vi "SetPiePlot.vi"(0 "reference in":refnum<class "HTMLPlot.lvclass">, 1 "PiePlot.PlotLabels":string[](array[string]), 2 "Dataset":dbl[][](array[numeric]), 3 "DatasetLabels":string[](array[string]), 5 "error in (no error)":errorcluster, 6 "DoughnutStyle":bool, 7 "PlotColours":u32[](array[colorbox])) -> (14 "reference out":refnum<class "HTMLPlot.lvclass">, 19 "error out":errorcluster)   [LabVIEW 2019, in "HTMLPlot.lvclass"]
uses:
  HTMLPlot.lvclass
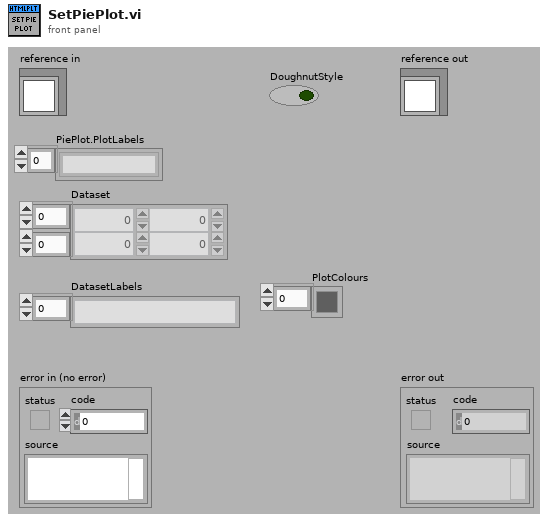
[diagram p1: front panel]
types:
  T1 = typedef "HTMLPlot.lvclass/ObjectAttributes.ctl" = cluster{"Attribute1":dbl, "GraphContainer":refnum<k7>, "ChartScriptFile":string, "UtilScriptFile(demoData)":string, "BaseHTML":string, "GenericProperties":cluster{"PlotType":T2, "PlotTitle":string, "XLabel":string, "YLabel":string, "ShowToolTip":bool}, "LegendProperties":cluster{"Show":bool, "Position":T3}, "BarPlot":cluster{"Dataset":dbl[][], "DatasetLabels":string[], "XLabels":string[], "PlotColours":u32[], "Stacked":bool}, "PiePlot":cluster{"Dataset":dbl[][], "DatasetLabels":string[], "PlotColours":u32[], "DoughnutStyle":bool, "PlotLabels":string[]}, "connection ID":refnum<k5>, "PortID":u64}
  T2 = typedef "HTMLPlot.lvclass/PlotType.ctl" = enum16{"bar", "line", "pie"}
  T3 = typedef "HTMLPlot.lvclass/LegendPosition.ctl" = enum16{"top", "right", "left", "bottom"}
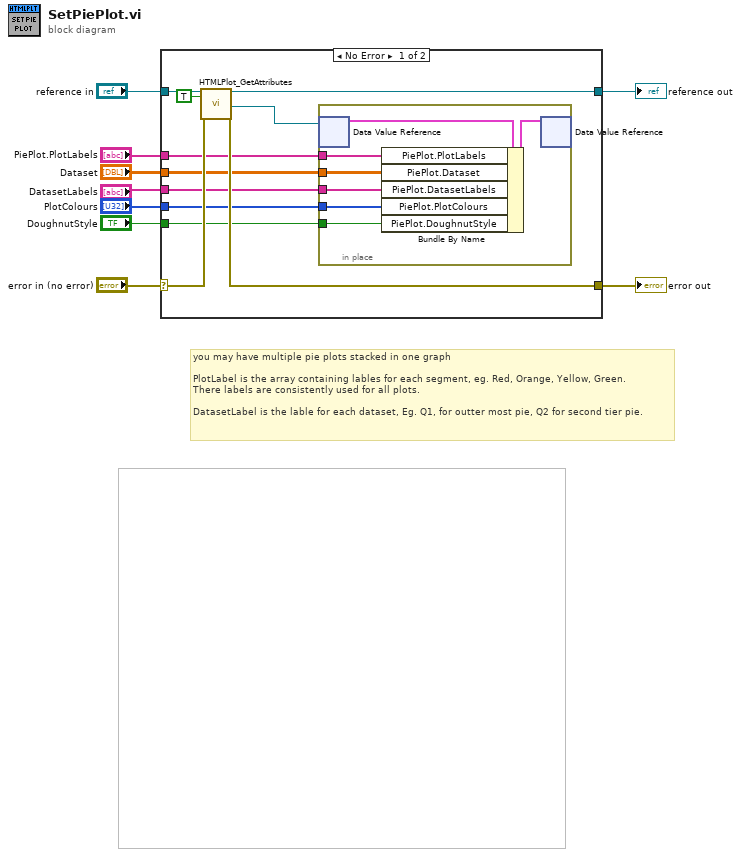
[diagram p0: block diagram]
diagram:
  # "you may have multiple pie plots stacked in one graph\n\nPlotLabel is the array containing lables for each segment, eg. Red, Orange, Yellow, Green.\nThere labels are consistently used for all plots.\n\nDatasetLabel is the lable for each dataset, Eg. Q1, for outter most pie, Q2 for second tier pie."
  n1 = case shown="No Error" "error in (no error)" {
    selector: "error in (no error)" -> [w20 w29]
    tunnel: [w19 w29] -> w8
    tunnel: [w17 w28] -> w6
    tunnel: "reference in" -> [w18 w28]
    tunnel: "Dataset" -> [w14 _]
    tunnel: "PlotColours" -> [w13 _]
    tunnel: "DatasetLabels" -> [w12 _]
    tunnel: "DoughnutStyle" -> [w11 _]
    tunnel: "PiePlot.PlotLabels" -> [w10 _]
    frame No Error {
      n2 = call "HTMLPlot_GetAttributes.vi"("reference in"=w18, "OnlyGetDvrReference(False)"=TRUE, "error in (no error)"=w20) -> ("reference out"=w17:refnum<class "HTMLPlot.lvclass">, "DataRef"=w15:refnum<data-value>, "error out"=w19:errorcluster)  [unwired: 13 in, 1 out]
      n3 = in-place {
        in-place-border: w14 -> [w27]
        in-place-border: w13 -> [w25]
        in-place-border: w12 -> [w23]
        in-place-border: w11 -> [w22]
        in-place-border: w10 -> [w21]
        n4 = in-place-dvr #1(w15) -> (w24:T1)  [unwired: 1 out]
        n5 = Bundle By Name(cluster=w24, "PiePlot.PlotLabels"=w21, "PiePlot.Dataset"=w27, "PiePlot.DatasetLabels"=w23, "PiePlot.PlotColours"=w25, "PiePlot.DoughnutStyle"=w22) -> (w26:T1)
        n6 = in-place-dvr #1(w26) -> ()  [unwired: 2 out]
      }
    }
    frame Error {
    }
  }
  "error out" <- w8
  "reference out" <- w6
